vi "Build Missing Tree Error.vi"(0 "Unique ID":string, 11 "Error In":errorcluster) -> (15 "Error Out":errorcluster)   [LabVIEW 2016, in "Tree Manager.lvclass"]
uses:
  Tree Manager.lvclass
  <vilib>/Utility/error.llb/Error Cluster From Error Code.vi
  <vilib>/ErrorRing/Error Ring.xnode
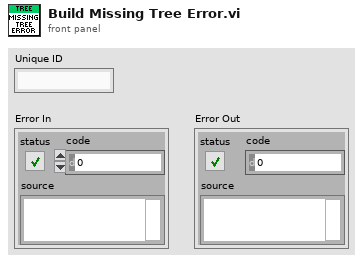
[diagram p1: front panel]
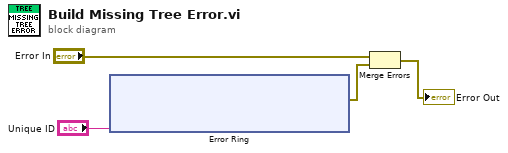
[diagram p0: block diagram]
diagram:
  n1 = xnode "Error Ring"("parameter 0"="Unique ID") -> ("error out"=w2:errorcluster)
  n2 = Merge Errors("Error In", w2) -> (→"Error Out":errorcluster)
